vi "Drive Keg Pump (V).vi"(8 "Error In":errorcluster, 11 "Voltage Select":i32) -> (0 "AO Error Out":errorcluster)   [LabVIEW 2020]
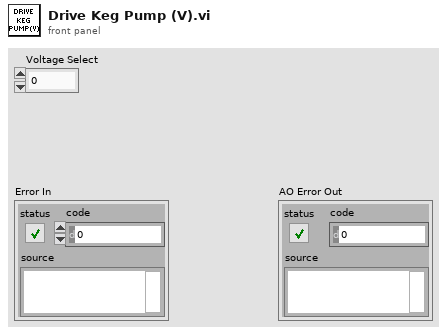
[diagram p1: front panel]
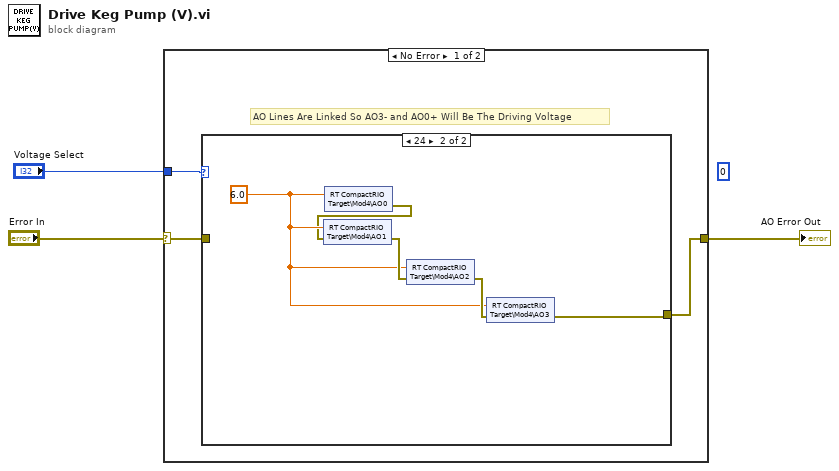
[diagram p0: block diagram]
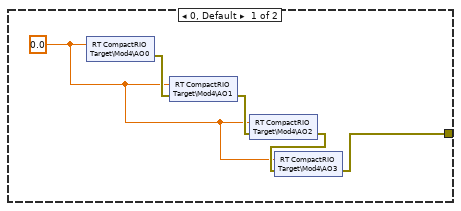
[diagram p2: hidden frame]
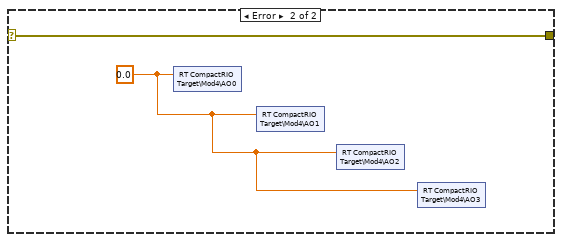
[diagram p3: hidden frame]
diagram:
  (unwired) 0 ("Voltage Select")
  n1 = case shown="No Error" "Error In" {
    selector: "Error In" -> [w4 w18]
    tunnel: "Voltage Select" -> [w6 _]
    tunnel: [w5 w18] -> w2
    frame No Error {
      # "AO Lines Are Linked So AO3- and AO0+ Will Be The Driving Voltage"
      n2 = case shown="24" w6 {
        tunnel: [w8 w14] -> w5
        tunnel: w4 -> [_ _]
        frame 0, Default {
          w7 = 0.0 ("AO0")
          n3 = shared-variable "RT CompactRIO Target\\Mod4\\AO0"(w7) -> (error out=w11:errorcluster)  [unwired: 1 in]
          n4 = shared-variable "RT CompactRIO Target\\Mod4\\AO1"(w7, error in=w11) -> (error out=w10:errorcluster)
          n5 = shared-variable "RT CompactRIO Target\\Mod4\\AO2"(w7, error in=w10) -> (error out=w9:errorcluster)
          n6 = shared-variable "RT CompactRIO Target\\Mod4\\AO3"(w7, error in=w9) -> (error out=w8:errorcluster)
        }
        frame 24 {
          w13 = 6.0 ("AO0")
          n7 = shared-variable "RT CompactRIO Target\\Mod4\\AO0"(w13) -> (error out=w12:errorcluster)  [unwired: 1 in]
          n8 = shared-variable "RT CompactRIO Target\\Mod4\\AO1"(w13, error in=w12) -> (error out=w15:errorcluster)
          n9 = shared-variable "RT CompactRIO Target\\Mod4\\AO2"(w13, error in=w15) -> (error out=w16:errorcluster)
          n10 = shared-variable "RT CompactRIO Target\\Mod4\\AO3"(w13, error in=w16) -> (error out=w14:errorcluster)
        }
      }
    }
    frame Error {
      w17 = 0.0 ("AO0")
      n11 = shared-variable "RT CompactRIO Target\\Mod4\\AO0"(w17) -> ()  [unwired: 1 in, 1 out]
      n12 = shared-variable "RT CompactRIO Target\\Mod4\\AO1"(w17) -> ()  [unwired: 1 in, 1 out]
      n13 = shared-variable "RT CompactRIO Target\\Mod4\\AO2"(w17) -> ()  [unwired: 1 in, 1 out]
      n14 = shared-variable "RT CompactRIO Target\\Mod4\\AO3"(w17) -> ()  [unwired: 1 in, 1 out]
    }
  }
  "AO Error Out" <- w2
